vi "ParseFlattenedData.vi"(0 "flattened data":u8[](array[numeric]), 1 "type descriptor":cluster{"TypeDescr":u8[], "Class":bool}[](array[cluster]), 2 "replace type desc":u8[](array[numeric]), 3 "type desc index":i32, 4 "replace object flatten data":u8[](array[numeric]), 5 "error in (no error)":errorcluster) -> (14 "element data":u8[](array[numeric]), 15 "remaining data":u8[](array[numeric]), 17 "type desc index out":i32, 18 "index out":i32[](array[numeric]), 19 "error out":errorcluster)   [LabVIEW 2020, in "G#DebugServer.lvclass"]
uses:
  G#DebugServer.lvclass
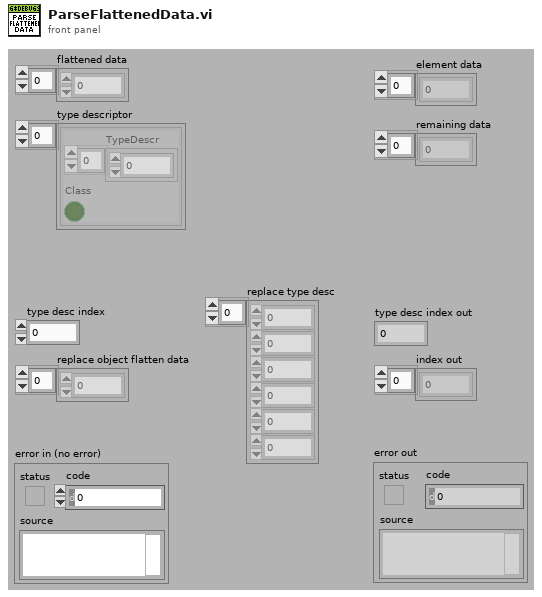
[diagram p1: front panel]
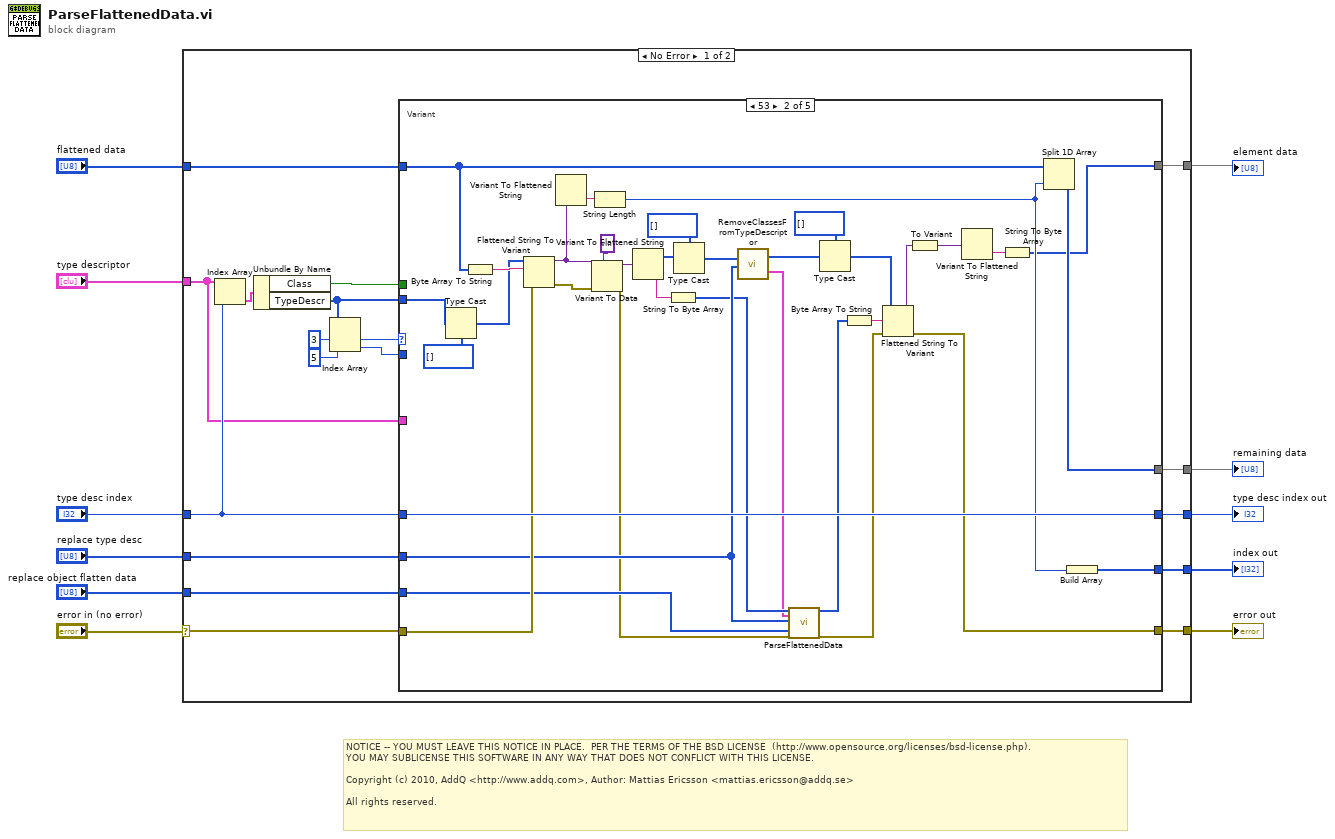
[diagram p0: block diagram]
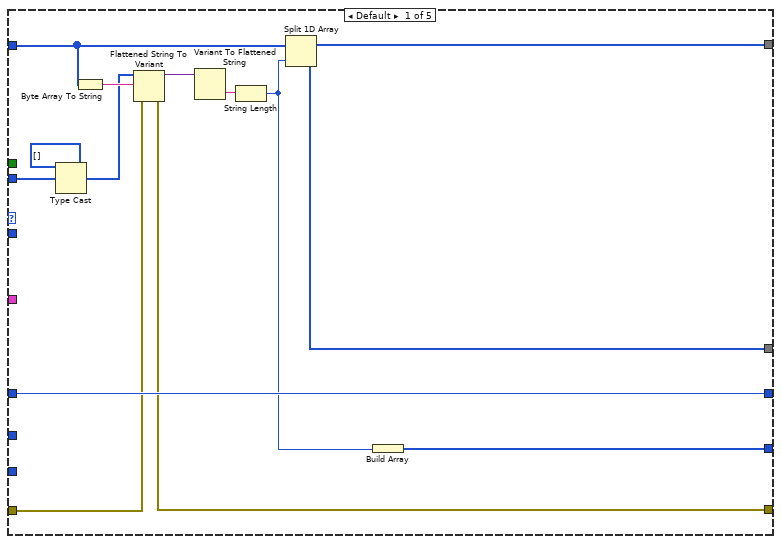
[diagram p2: hidden frame]
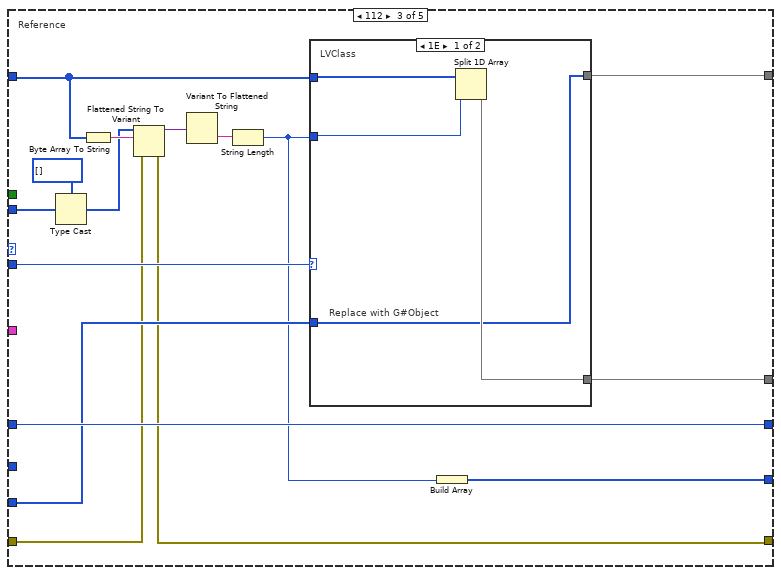
[diagram p3: hidden frame]
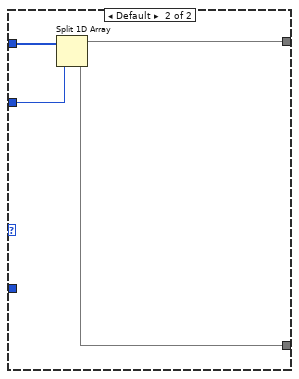
[diagram p4: hidden frame]
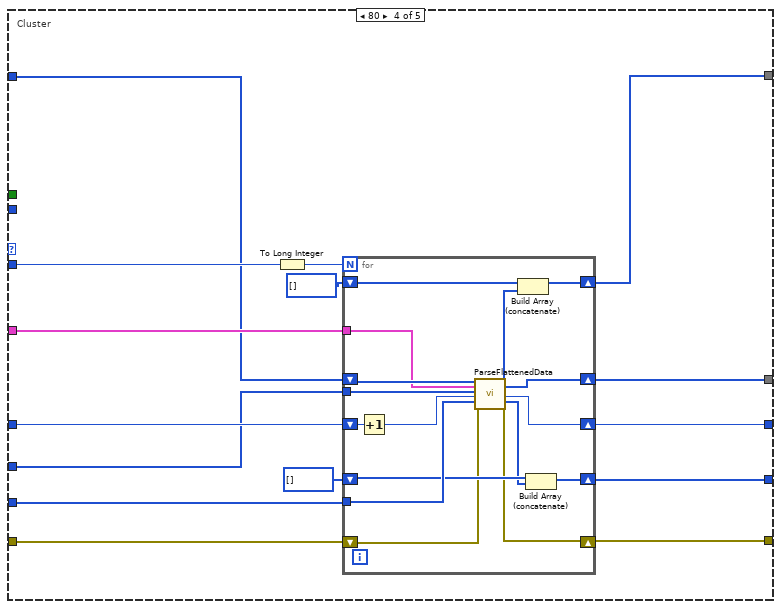
[diagram p5: hidden frame]
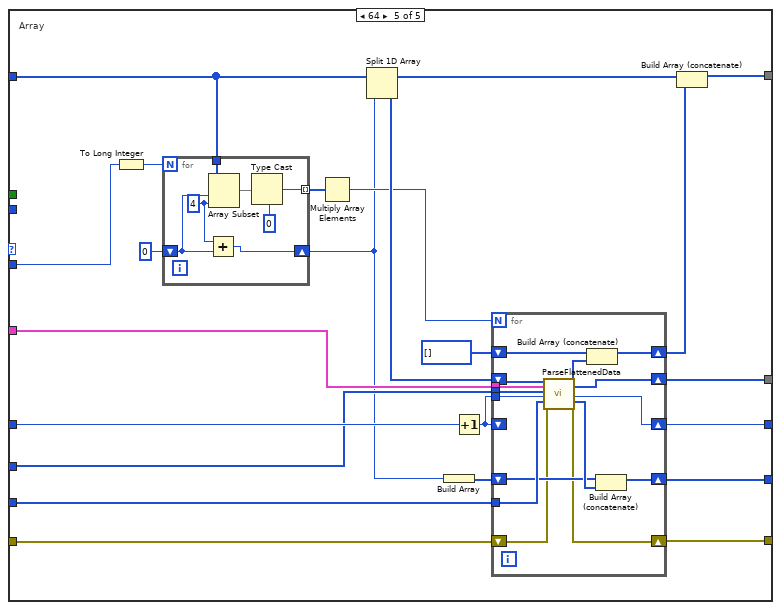
[diagram p6: hidden frame]
diagram:
  # "NOTICE -- YOU MUST LEAVE THIS NOTICE IN PLACE.  PER THE TERMS OF THE BSD LICENSE  (http://www.opensource.org/licenses/bsd-license.php).\nYOU MAY SUBLICENSE THIS SOFTWARE IN ANY WAY THAT DOES NOT CONFLICT WITH THIS LICENSE.\n\nCopyright (c) 2010, AddQ <http://www.addq.com>, Author: Mattias Ericsson <mattias.ericsson@addq.se>\n\nAll rights reserved."
  n1 = case shown="No Error" "error in (no error)" {
    selector: "error in (no error)" -> [w18 w180]
    tunnel: "flattened data" -> [w29 _]
    tunnel: "replace object flatten data" -> [w28 _]
    tunnel: [w27 _] -> w9
    tunnel: "type desc index" -> [w26 w179]
    tunnel: [w25 w179] -> w7
    tunnel: [w24 _] -> w6
    tunnel: [w23 _] -> w5
    tunnel: "type descriptor" -> [w22 _]
    tunnel: [w21 w180] -> w3
    tunnel: "replace type desc" -> [w19 _]
    frame No Error {
      n2 = Index Array(array=w22, index=w26) -> (element=w20:cluster{"TypeDescr":u8[], "Class":bool})
      n3 = Unbundle By Name(w20) -> ("Class"=w12:bool, "TypeDescr"=w17:u8[])
      n4 = Index Array(array=w17, index #1=3 ("index"), index #2=5 ("index")) -> (element #1=w14:u8, element #2=w13:u8)
      n5 = case shown="53" w14 {
        tunnel: w13 -> [_ _ w84 w117 w156]
        tunnel: w17 -> [w42 w77 w81 _ _]
        tunnel: w22 -> [_ _ _ w116 w147]
        tunnel: w26 -> [w36 w74 w88 w115 w154]
        tunnel: w28 -> [_ w62 w83 w114 w153]
        tunnel: w29 -> [w37 w75 w89 w113 w155]
        tunnel: [w33 w72 w85 w112 w152] -> w23
        tunnel: [w36 w74 w88 w111 w145] -> w25
        tunnel: [w35 w68 w87 w110 w150] -> w24
        tunnel: [w34 w73 w86 w109 w151] -> w27
        tunnel: w18 -> [w31 w71 w82 w108 w149]
        tunnel: [w30 w65 w79 w107 w148] -> w21
        tunnel: w19 -> [_ w63 _ w106 w146]
        tunnel: w12 -> [_ _ _ _ _]
        frame Default {
          n6 = Type Cast(type=i16[] [] ("TypeDescr"), x=w42) -> (*(type *) &x=w40:i16[])
          n7 = Byte Array To String(unsigned byte array=w37) -> (string=w43:string)
          n8 = Flattened String To Variant(4:w31, 6:w43, 7:w40) -> (0:w30:errorcluster, 3:w39:variant)
          n9 = Variant To Flattened String(Variant=w39) -> (data string=w38:string)  [unwired: 1 out]
          n10 = String Length(string=w38) -> (length=w32:i32)
          n11 = Split 1D Array(array=w37, index=w32) -> (first subarray=w35:u8[], second subarray=w34:u8[])
          n12 = Build Array(w32) -> (w33:i32[])
        }
        frame 83 {
          # "Variant"
          n13 = Type Cast(type=i16[] [] ("TypeDescr"), x=w77) -> (*(type *) &x=w60:i16[])
          n14 = Byte Array To String(unsigned byte array=w75) -> (string=w78:string)
          n15 = Flattened String To Variant(4:w71, 6:w78, 7:w60) -> (0:w67:errorcluster, 3:w66:variant)
          n16 = Variant To Flattened String(Variant=w66) -> (data string=w70:string)  [unwired: 1 out]
          n17 = Variant To Data(error in=w67, type=variant, Variant=w66) -> (data=w59:variant, error out=w53:errorcluster)
          n18 = String Length(string=w70) -> (length=w69:i32)
          n19 = Variant To Flattened String(Variant=w59) -> (data string=w52:string, 1:w58:i16[])
          n20 = String To Byte Array(string=w52) -> (unsigned byte array=w51:u8[])
          n21 = Type Cast(type=u8[] [] ("TypeDescr"), x=w58) -> (*(type *) &x=w56:u8[])
          n22 = call "RemoveClassesFromTypeDescriptor.vi"("type descriptor"=w56, "replace type desc"=w63) -> ("type descriptor out"=w54:u8[], "type descriptor parsed out"=w50:cluster{"TypeDescr":u8[], "Class":bool}[])  [unwired: 16 in]
          n23 = call "ParseFlattenedData.vi"("flattened data"=w51, "type descriptor"=w50, "replace type desc"=w63, "replace object flatten data"=w62, "error in (no error)"=w53) -> ("element data"=w47:u8[], "error out"=w49:errorcluster)  [unwired: 10 in, 3 out]
          n24 = Type Cast(type=i16[] [] ("TypeDescr"), x=w54) -> (*(type *) &x=w44:i16[])
          n25 = Byte Array To String(unsigned byte array=w47) -> (string=w48:string)
          n26 = Flattened String To Variant(4:w49, 6:w48, 7:w44) -> (0:w65:errorcluster, 3:w46:variant)
          n27 = To Variant(anything=w46) -> (Variant=w61:variant)
          n28 = Variant To Flattened String(Variant=w61) -> (data string=w64:string)  [unwired: 1 out]
          n29 = String To Byte Array(string=w64) -> (unsigned byte array=w68:u8[])
          n30 = Split 1D Array(array=w75, index=w69) -> (second subarray=w73:u8[])  [unwired: 1 out]
          n31 = Build Array(w69) -> (w72:i32[])
        }
        frame 112 {
          # "Reference"
          n32 = Type Cast(type=i16[] [] ("TypeDescr"), x=w81) -> (*(type *) &x=w92:i16[])
          n33 = Byte Array To String(unsigned byte array=w89) -> (string=w94:string)
          n34 = Flattened String To Variant(4:w82, 6:w94, 7:w92) -> (0:w79:errorcluster, 3:w91:variant)
          n35 = Variant To Flattened String(Variant=w91) -> (data string=w90:string)  [unwired: 1 out]
          n36 = String Length(string=w90) -> (length=w80:i32)
          n37 = case shown="1E" w84 {
            tunnel: w89 -> [w96 w102]
            tunnel: [w95 w101] -> w87
            tunnel: [w98 w100] -> w86
            tunnel: w80 -> [w97 w99]
            tunnel: w83 -> [w95 _]
            frame 30 {
              # "Replace with G#Object"
              # "LVClass"
              n38 = Split 1D Array(array=w96, index=w97) -> (second subarray=w98:u8[])  [unwired: 1 out]
            }
            frame Default {
              n39 = Split 1D Array(array=w102, index=w99) -> (first subarray=w101:u8[], second subarray=w100:u8[])
            }
          }
          n40 = Build Array(w80) -> (w85:i32[])
        }
        frame 80 {
          # "Cluster"
          n41 = To Long Integer(number=w117) -> (32bit integer=w103:i32)
          n42 = for {
            N: w103 -> [_]
            shift-right: [w131] -> w110
            shift-left: u8[] [] -> [w130]
            shift-right: [w133] -> w109
            shift-left: w113 -> [w132]
            tunnel: w114 -> [w127]
            shift-right: [w126] -> w111
            shift-left: w115 -> [w128]
            shift-right: [w122] -> w112
            shift-left: i32[] [] -> [w124]
            tunnel: w116 -> [w121]
            tunnel: w106 -> [w118]
            shift-right: [w119] -> w107
            shift-left: w108 -> [w120]
            n43 = Increment(x=w128) -> (x+1=w125:i32)
            n44 = call "ParseFlattenedData.vi"("flattened data"=w132, "type descriptor"=w121, "replace type desc"=w118, "type desc index"=w125, "replace object flatten data"=w127, "error in (no error)"=w120) -> ("element data"=w129:u8[], "remaining data"=w133:u8[], "type desc index out"=w126:i32, "index out"=w123:i32[], "error out"=w119:errorcluster)  [unwired: 9 in]
            n45 = Build Array (concatenate)(w130, w129) -> (w131:u8[])
            n46 = Build Array (concatenate)(w124, w123) -> (w122:i32[])
          }
        }
        frame 64 {
          # "Array"
          n47 = To Long Integer(number=w156) -> (32bit integer=w135:i32)
          n48 = for {
            N: w135 -> [_]
            tunnel: w155 -> [w176]
            tunnel: [w175] -> w144 mode=indexing
            shift-right: [w172] -> w137
            shift-left: 0 -> [w173]
            w174 = 4 ("length")
            n49 = Add(x=w174, y=w173) -> (x+y=w172:i32)
            n50 = Array Subset(array=w176, index=w173, length=w174) -> (w178:u8[])
            n51 = Type Cast(type=0, x=w178) -> (*(type *) &x=w175:i32)
          }
          n52 = Multiply Array Elements(1:w144) -> (0:w140:i32)
          n53 = Split 1D Array(array=w155, index=w137) -> (first subarray=w139:u8[], second subarray=w142:u8[])
          n54 = Build Array(w137) -> (w138:i32[])
          n55 = Increment(x=w154) -> (x+1=w134:i32)
          n56 = for {
            N: w140 -> [_]
            shift-right: [w169] -> w136
            shift-left: u8[] [] ("second subarray") -> [w168]
            shift-right: [w171] -> w151
            shift-left: w142 -> [w170]
            tunnel: w153 -> [w165]
            shift-right: [w162] -> w152
            shift-left: w138 -> [w163]
            tunnel: w147 -> [w159]
            tunnel: w146 -> [w158]
            shift-right: [w160] -> w148
            shift-left: w149 -> [w161]
            tunnel: w134 -> [w166]
            shift-right: [w157] -> w145
            shift-left: w134 -> [_]
            n57 = call "ParseFlattenedData.vi"("flattened data"=w170, "type descriptor"=w159, "replace type desc"=w158, "type desc index"=w166, "replace object flatten data"=w165, "error in (no error)"=w161) -> ("element data"=w167:u8[], "remaining data"=w171:u8[], "type desc index out"=w157:i32, "index out"=w164:i32[], "error out"=w160:errorcluster)  [unwired: 9 in]
            n58 = Build Array (concatenate)(w168, w167) -> (w169:u8[])
            n59 = Build Array (concatenate)(w163, w164) -> (w162:i32[])
          }
          n60 = Build Array (concatenate)(w139, w136) -> (w150:u8[])
        }
      }
    }
    frame Error {
    }
  }
  "remaining data" <- w9
  "type desc index out" <- w7
  "element data" <- w6
  "index out" <- w5
  "error out" <- w3
